vi "CollectorWrap.vi"(7 "Action":T1=enum."Collect", 8 "error in":errorcluster) -> (0 "error out":errorcluster, 2 "StateOut":T1, 3 "Enque?":bool)   [LabVIEW 2013]
uses:
  DoubleSolenoidAction.ctl
  RollerAction.ctl
  CollectorWrapAction.ctl
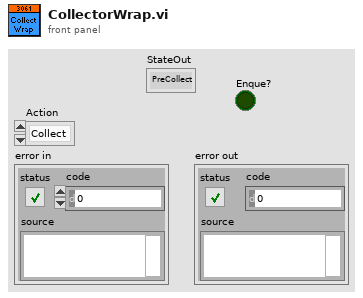
[diagram p1: front panel]
types:
  T1 = typedef "CollectorWrapAction.ctl" = enum16{"PreCollect", "Collect", "Stop"}
  T2 = typedef "DoubleSolenoidAction.ctl" = enum16{"Init", "Middle", "In", "Out"}
  T3 = typedef "RollerAction.ctl" = enum16{"Init", "Off", "Forward", "Reverse"}
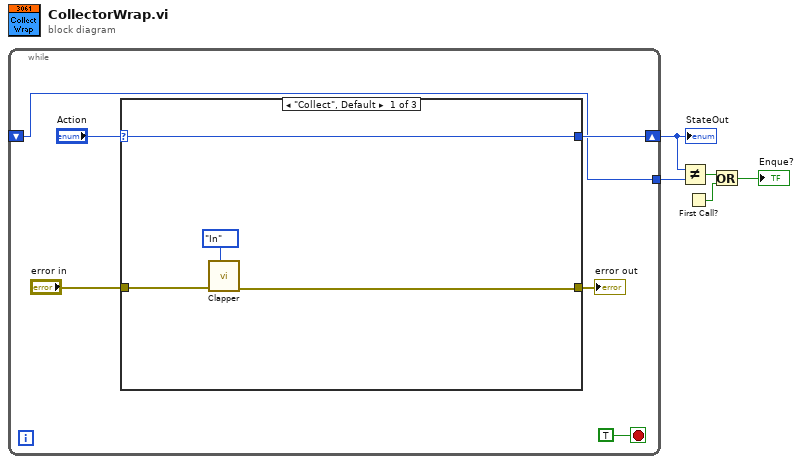
[diagram p0: block diagram]
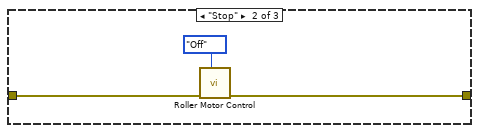
[diagram p2: hidden frame]
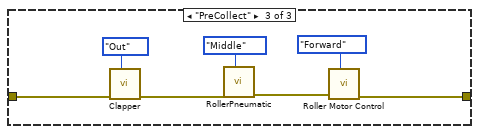
[diagram p3: hidden frame]
diagram:
  n1 = while {
    shift-right: [w7] -> w5
    shift-left: _ -> [w6]
    tunnel: [w6] -> w4
    stop <- TRUE stop-if-true
    n2 = case shown="\"Collect\", Default" "Action" {
      selector: "Action" -> [w12 _ _]
      tunnel: "error in" -> [w15 w18 w23]
      tunnel: [w14 w17 w25] -> w8
      tunnel: [w12 _ _] -> w7
      frame "Collect", Default {
        n3 = call "Clapper.vi"("State"=DoubleSolenoidAction."In", "Error in"=w15) -> ("Error out"=w14:errorcluster)  [unwired: 9 in]
      }
      frame "Stop" {
        n4 = call "Roller Motor Control.vi"("Action"=RollerAction."Off", "Error in"=w18) -> ("Error out"=w17:errorcluster)  [unwired: 9 in]
      }
      frame "PreCollect" {
        n5 = call "Clapper.vi"("State"=DoubleSolenoidAction."Out", "Error in"=w23) -> ("Error out"=w22:errorcluster)  [unwired: 9 in]
        n6 = call "RollerPneumatic.vi"("State"=DoubleSolenoidAction."Middle", "Error in"=w22) -> ("Error out"=w21:errorcluster)  [unwired: 9 in]
        n7 = call "Roller Motor Control.vi"("Action"=RollerAction."Forward", "Error in"=w21) -> ("Error out"=w25:errorcluster)  [unwired: 9 in]
      }
    }
    "error out" <- w8
  }
  "StateOut" <- w5
  n8 = Not Equal?(x=w5, y=w4) -> (x != y?=w3:bool)
  n9 = First Call?() -> (First Call?: T/F=w2:bool)
  n10 = Or(x=w3, y=w2) -> (x .or. y?=→"Enque?":bool)
